vi "Mosi Logic 64-bit.vi"(0 "data to send":u64 format="%.0x", 5 "transfer settings":T2 {"Direction Change Bit" max=64 step=1; "Transfer Length (bits)" min=1 max=64 step=1}, 7 "controller interface":T1, 9 "shift MOSI":bool) -> (4 "MOSI":bool, 6 "MOSI enable":bool)   [LabVIEW 2015, in "SPI API.lvlib"]
doc: "This VI controls shifting MOSI data out of the FPGA."
uses:
  <userlib>/_NI SPI IP/FPGA/Controllers/Public/Transfer Settings.ctl
  Controls/Controller Interface.ctl
  SPI API.lvlib
  <userlib>/_NI SPI IP/FPGA/Controllers/NI SPI IP FPGA.lvlib
panel:
  # "This VI controls shifting MOSI data out of the FPGA."
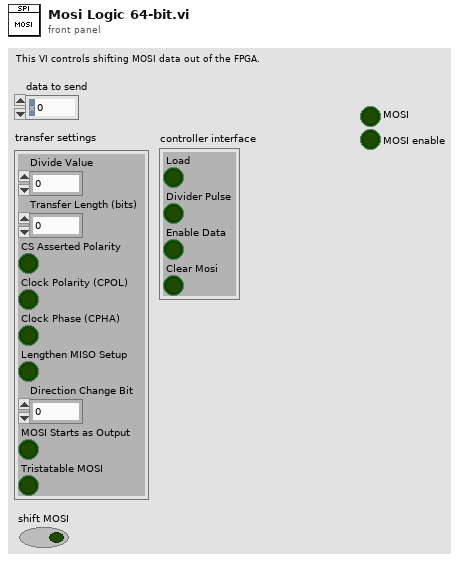
[diagram p1: front panel]
types:
  T1 = typedef "SPI API.lvlib/Controller Interface.ctl" = cluster{"Load":bool, "Divider Pulse":bool, "Enable Data":bool, "Clear Mosi":bool}
  T2 = typedef "NI SPI IP FPGA.lvlib/Transfer Settings.ctl" = cluster{"Divide Value":u8, "Transfer Length (bits)":u8, "CS Asserted Polarity":bool, "Clock Polarity (CPOL)":bool, "Clock Phase (CPHA)":bool, "Lengthen MISO Setup":bool, "Direction Change Bit":u8, "MOSI Starts as Output":bool, "Tristatable MOSI":bool}
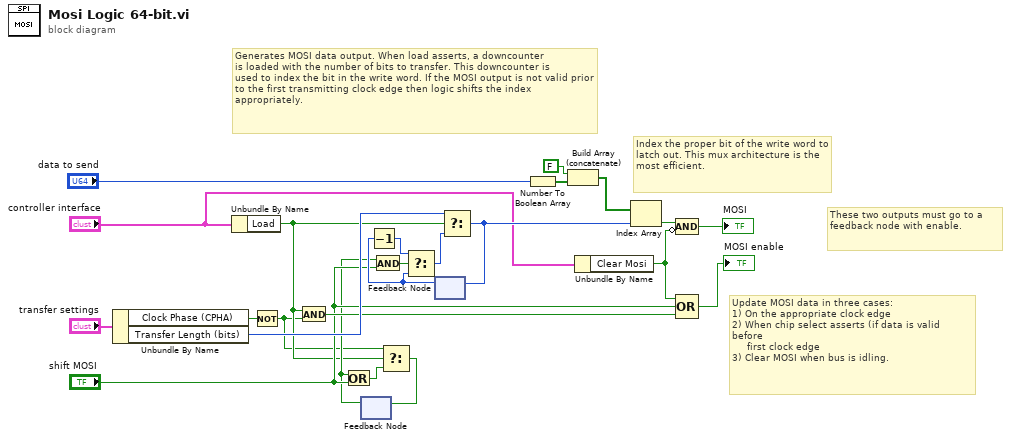
[diagram p0: block diagram]
diagram:
  # "These two outputs must go to a feedback node with enable."
  # "Generates MOSI data output. When load asserts, a downcounter\nis loaded with the number of bits to transfer. This downcounter is\nused to index the bit in the write word. If the MOSI output is not valid prior to the first transmitting clock edge then logic shifts the index appropriately."
  # "Update MOSI data in three cases:\n1) On the appropriate clock edge\n2) When chip select asserts (if data is valid before\n     first clock edge\n3) Clear MOSI when bus is idling."
  # "Index the proper bit of the write word to latch out. This mux architecture is the most efficient."
  n1 = Unbundle By Name("transfer settings") -> ("Clock Phase (CPHA)"=w5:bool, "Transfer Length (bits)"=w13:u8)
  n2 = Unbundle By Name("controller interface") -> ("Load"=w6:bool)
  n3 = Not(x=w5) -> (.not. x?=w4:bool)
  n4 = And(x=w6, y=w4) -> (x .and. y?=w12:bool)
  n5 = feedback #1() -> (w8:bool)  [unwired: 1 in]
  n6 = Or(x=w8, y="shift MOSI") -> (x .or. y?=w11:bool)
  n7 = And(x=w8, y="shift MOSI") -> (x .and. y?=w7:bool)
  n8 = Select(t=w4, s=w6, f=w11) -> (s? t:f=w10:bool)
  n9 = feedback-in #1(w10) -> ()
  n10 = feedback #2() -> (w22:u8)  [unwired: 1 in]
  n11 = Decrement(x=w22) -> (x-1=w24:u8)
  n12 = Select(t=w24, s=w7, f=w22) -> (s? t:f=w23:u8)
  n13 = Select(t=w13, s=w6, f=w23) -> (s? t:f=w18:u8)
  n14 = feedback-in #2(w18) -> ()
  n15 = Number To Boolean Array(number="data to send") -> (Boolean array=w19:bool[])
  n16 = Build Array (concatenate)(FALSE, w19) -> (w17:bool[])
  n17 = Unbundle By Name("controller interface") -> ("Clear Mosi"=w16:bool)
  n18 = Index Array(array=w17, index=w18) -> (element=w21:bool)
  n19 = Compound Arithmetic op=AND(w21, invert w16) -> (→"MOSI":bool)
  n20 = Compound Arithmetic op=OR(w16, "shift MOSI", w12) -> (→"MOSI enable":bool)
